vi "motor-position-query-v2.vi"(8 "error in (no error)":errorcluster, 10 "Unit":enum16{"fs", "ps", "um", "mm", "counts"}(ring), 11 "Axis Select":u8(slide)=1 min=1 max=4 scale=1.0..4.0) -> (0 "error out":errorcluster, 1 "Initial Position of motor":string, 2 "Initial Position in selected unit":dbl, 3 "Initial Position in counts":dbl)   [LabVIEW 2009]
doc: "This VI provides the current position of PI stage in selected unit as well as the machine language counts and a string for position with unit."
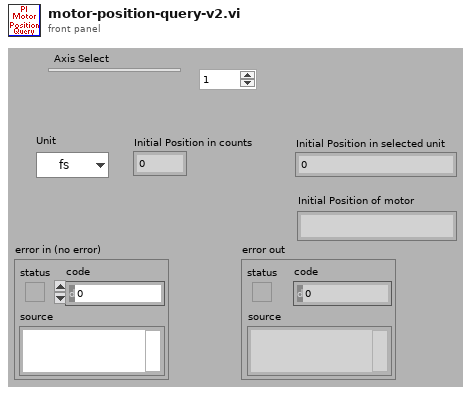
[diagram p1: front panel]
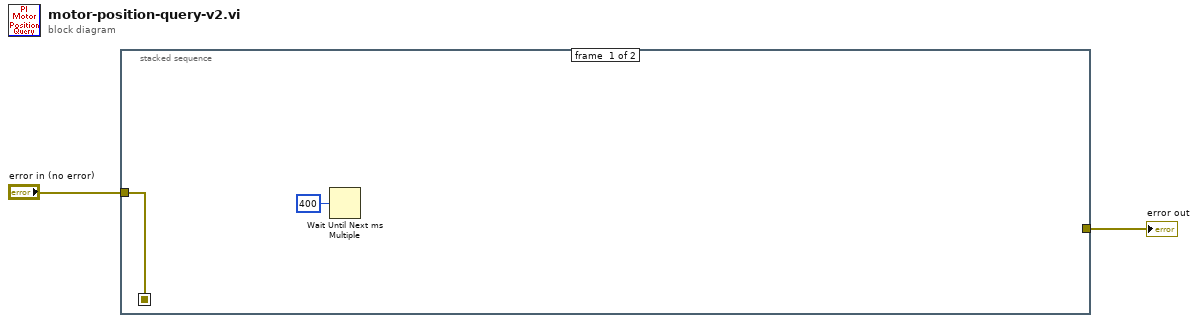
[diagram p0: block diagram]
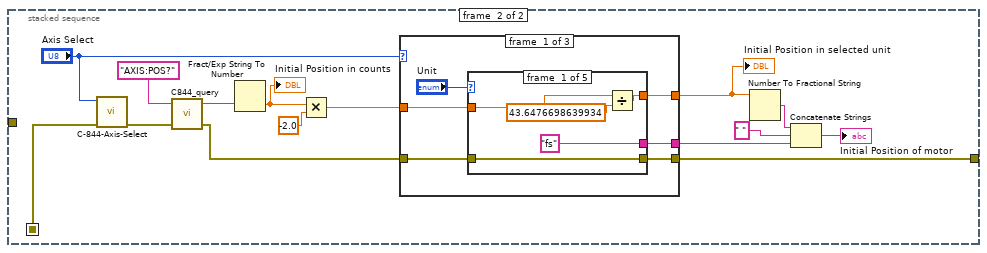
[diagram p2: hidden frame]
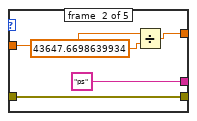
[diagram p3: hidden frame]
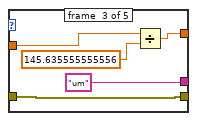
[diagram p4: hidden frame]
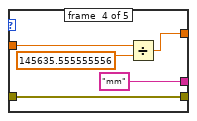
[diagram p5: hidden frame]
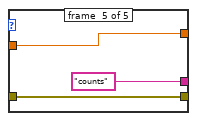
[diagram p6: hidden frame]
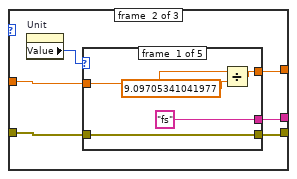
[diagram p7: hidden frame]
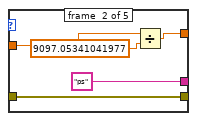
[diagram p8: hidden frame]
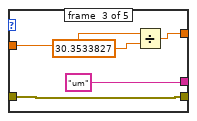
[diagram p9: hidden frame]
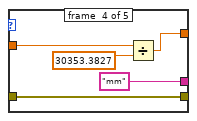
[diagram p10: hidden frame]
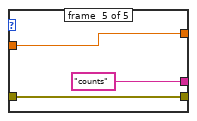
[diagram p11: hidden frame]
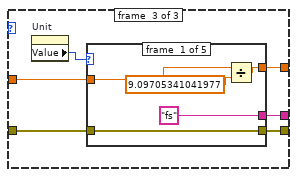
[diagram p12: hidden frame]
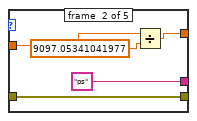
[diagram p13: hidden frame]
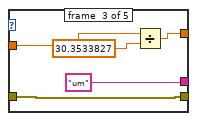
[diagram p14: hidden frame]
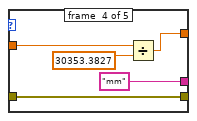
[diagram p15: hidden frame]
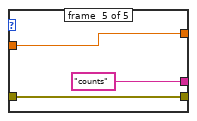
[diagram p16: hidden frame]
diagram:
  n1 = stacked-sequence {
    seq-local: [w3 _] -> [_ w9]
    tunnel: "error in (no error)" -> [w3 _]
    tunnel: [_ w6] -> w1
    frame #0 {
      n2 = Wait Until Next ms Multiple(millisecond multiple=u32 400) -> ()  [unwired: 1 out]
    }
    frame #1 {
      n3 = call "C-844-Axis-Select.vi"("error in (no error)"=w9, "Axis Select"="Axis Select") -> ("error out"=w10:errorcluster)  [unwired: 8 in, 1 out]
      n4 = call "C844_query.vi"("Error in"=w10, "Command"="AXIS:POS?") -> ("Error out"=w7:errorcluster, "Response"=w19:string)  [unwired: 2 in]
      n5 = Fract/Exp String To Number(string=w19) -> (number=w13:dbl)  [unwired: 3 in, 1 out]
      "Initial Position in counts" <- w13
      n6 = Multiply(x=w13, y=-2.0) -> (x*y=w11:dbl)
      n7 = case shown="1, Default" "Axis Select" {
        tunnel: [w24 w52 w81] -> w14
        tunnel: w11 -> [w23 w54 w83]
        tunnel: [w22 w51 w80] -> w8
        tunnel: w7 -> [w21 w53 w82]
        tunnel: [w20 w50 w79] -> w6
        frame #0 {
          n8 = case shown="\"counts\"" "Unit" {
            tunnel: w23 -> [w29 w34 w39 w44 w48]
            tunnel: [w28 w33 w38 w43 w48] -> w24
            tunnel: ["fs" "ps" "um" "mm" "counts"] -> w22
            tunnel: w21 -> [w26 w31 w36 w41 w46]
            tunnel: [w26 w31 w36 w41 w46] -> w20
            frame #0 {
              n9 = Divide(x=w29, y=43.6476698639934) -> (x/y=w28:dbl)
            }
            frame #1 {
              n10 = Divide(x=w34, y=43647.6698639934) -> (x/y=w33:dbl)
            }
            frame #2 {
              n11 = Divide(x=w39, y=145.635555555556) -> (x/y=w38:dbl)
            }
            frame #3 {
              n12 = Divide(x=w44, y=145635.555555556) -> (x/y=w43:dbl)
            }
            frame #4 {
            }
          }
        }
        frame #1 {
          n13 = property on="Unit" class="Enum (strict)"() -> ("Value"=w49:enum16{"fs", "ps", "um", "mm", "counts"})  [unwired: 2 in, 2 out]
          n14 = case shown="\"fs\", Default" w49 {
            tunnel: w54 -> [w58 w63 w68 w73 w77]
            tunnel: [w57 w62 w67 w72 w77] -> w52
            tunnel: ["fs" "ps" "um" "mm" "counts"] -> w51
            tunnel: w53 -> [w55 w60 w65 w70 w75]
            tunnel: [w55 w60 w65 w70 w75] -> w50
            frame #0 {
              n15 = Divide(x=w58, y=9.09705341041977) -> (x/y=w57:dbl)
            }
            frame #1 {
              n16 = Divide(x=w63, y=9097.05341041977) -> (x/y=w62:dbl)
            }
            frame #2 {
              n17 = Divide(x=w68, y=30.3533827) -> (x/y=w67:dbl)
            }
            frame #3 {
              n18 = Divide(x=w73, y=30353.3827) -> (x/y=w72:dbl)
            }
            frame #4 {
            }
          }
        }
        frame #2 {
          n19 = property on="Unit" class="Enum (strict)"() -> ("Value"=w78:enum16{"fs", "ps", "um", "mm", "counts"})  [unwired: 2 in, 2 out]
          n20 = case shown="\"mm\"" w78 {
            tunnel: w83 -> [w87 w92 w97 w102 w106]
            tunnel: [w86 w91 w96 w101 w106] -> w81
            tunnel: ["fs" "ps" "um" "mm" "counts"] -> w80
            tunnel: w82 -> [w84 w89 w94 w99 w104]
            tunnel: [w84 w89 w94 w99 w104] -> w79
            frame #0 {
              n21 = Divide(x=w87, y=9.09705341041977) -> (x/y=w86:dbl)
            }
            frame #1 {
              n22 = Divide(x=w92, y=9097.05341041977) -> (x/y=w91:dbl)
            }
            frame #2 {
              n23 = Divide(x=w97, y=30.3533827) -> (x/y=w96:dbl)
            }
            frame #3 {
              n24 = Divide(x=w102, y=30353.3827) -> (x/y=w101:dbl)
            }
            frame #4 {
            }
          }
        }
      }
      "Initial Position in selected unit" <- w14
      n25 = Number To Fractional String(number=w14) -> (F-format string=w17:string)  [unwired: 3 in]
      n26 = Concatenate Strings(w17, " ", w8) -> (→"Initial Position of motor":string)
    }
  }
  "error out" <- w1
